vi "test Compare Labels.vi"(8 "error in":errorcluster, 11 "TestCase in":refnum<class "Refresh.lvclass">) -> (0 "error out":errorcluster, 3 "TestCase out":refnum<class "Refresh.lvclass">)   [LabVIEW 2020, in "Refresh.lvclass"]
uses:
  Refresh.lvclass
  <vilib>/addons/_JKI Toolkits/VI Tester/TestCase.llb/TestCase.lvclass
  Encoding and Decoding/Encoding.ctl
  Encoding and Decoding/Encoding and Decoding.lvlib
  Shared/Parameter Definition.ctl
  Shared/VS Channel Definition for Parameter.ctl
  System Explorer/Implementation/System Explorer/Types/Refresh Symbols.ctl
  System Explorer/Implementation/Implementation.lvlib
  System Explorer/Implementation/System Explorer/Types/Refresh Listbox.ctl
  Shared/Transfer Type.ctl
  Shared/VS Channels Definition for Label.ctl
  C:/Program Files (x86)/National Instruments/LabVIEW 2020/vi.lib/addons/_JKI Toolkits/VI Tester/TestCase.llb/TestCase.lvclass
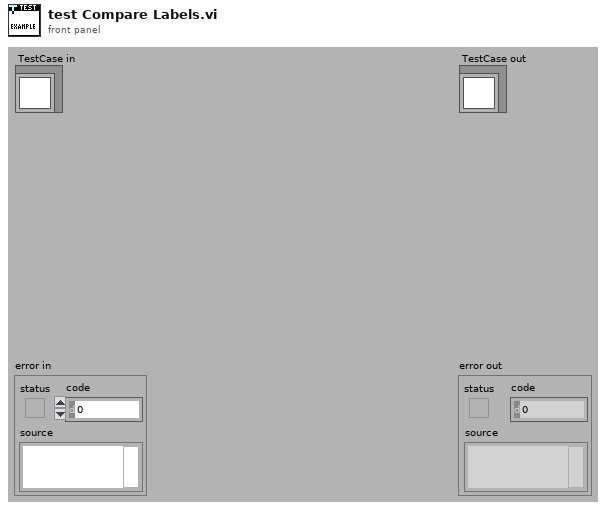
[diagram p1: front panel]
types:
  T1 = typedef "Ballard ARINC 429 System Explorer.lvlib/Implementation.lvlib/Refresh Listbox.ctl" = cluster{"Item Names":string[], "Item Symbol":T2, "Change Flag":bool}
  T2 = typedef "Ballard ARINC 429 System Explorer.lvlib/Implementation.lvlib/Refresh Symbols.ctl" = enum16{"Blank", "Port", "Incoming", "Outgoing", "Label", "Word", "Parameter", "ARINC-429", "Config Files", "Channel Spec", "Item"}
  T3 = typedef "VS Channels Definition for Label.ctl" = cluster{"label (Dec)":u32, "parameters":T4[], "SDI value":u8, "SDI enabled":bool, "transfer type":T7, "create timestamp":bool}
  T4 = typedef "VS Channel Definition for Parameter.ctl" = cluster{"name":string, "default value":dbl, "unit":string, "Parameter":T5}
  T5 = typedef "Parameter Definition.ctl" = cluster{"start index":i32, "size":i32, "encoding":T6, "signed":bool, "scale multiplier":dbl, "scale offset":dbl}
  T6 = typedef "Encoding and Decoding.lvlib/Encoding.ctl" = enum16{"BNR", "BCD", "Discrete"}
  T7 = typedef "Transfer Type.ctl" = enum16{"Scheduled", "Acyclic", "Block", "Strobe"}
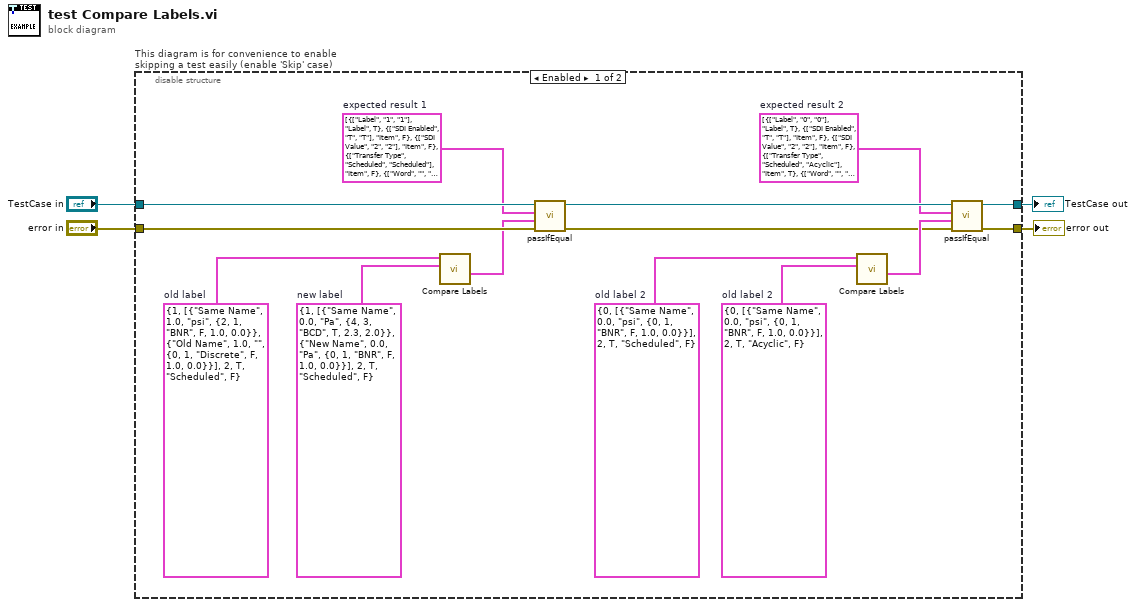
[diagram p0: block diagram]
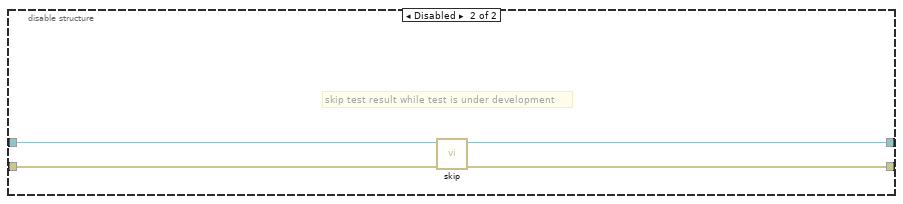
[diagram p2: hidden frame]
diagram:
  n1 = disable-structure "This diagram is for convenience to enable skipping a test easily (enable 'Skip' case)" shown="Enabled" {
    disable-tunnel: "TestCase in" -> [w18 w19]
    disable-tunnel: [w9 w20] -> w1
    disable-tunnel: [w8 w22] -> w3
    disable-tunnel: "error in" -> [w17 w21]
    frame Enabled {
      w5 = T1[] [{"Item Names"=["Label", "0", "0"], "Item Symbol"=enum."Label", "Change Flag"=TRUE}, {"Item Names"=["SDI Enabled", "TRUE", "TRUE"], "Item Symbol"=enum."Item", "Change Flag"=FALSE}, {"Item Names"=["SDI Value", "2", "2"], "Item Symbol"=enum."Item", "Change Flag"=FALSE}, {"Item Names"=["Transfer Type", "Scheduled", "Acyclic"], "Item Symbol"=enum."Item", "Change Flag"=TRUE}, {"Item Names"=["Word", "", ""], "Item Symbol"=enum."Word", "Change Flag"=FALSE}, {"Item Names"=["Parameter", "Same Name", "Same Name"], "Item Symbol"=enum."Parameter", "Change Flag"=FALSE}, {"Item Names"=["Encoding", "BNR", "BNR"], "Item Symbol"=enum."Item", "Change Flag"=FALSE}, {"Item Names"=["Default Value", "0.000000", "0.000000"], "Item Symbol"=enum."Item", "Change Flag"=FALSE}, {"Item Names"=["Start Index", "0", "0"], "Item Symbol"=enum."Item", "Change Flag"=FALSE}, {"Item Names"=["Size", "1", "1"], "Item Symbol"=enum."Item", "Change Flag"=FALSE}, {"Item Names"=["Signed", "FALSE", "FALSE"], "Item Symbol"=enum."Item", "Change Flag"=FALSE}, {"Item Names"=["Scale Factor", "1.000000", "1.000000"], "Item Symbol"=enum."Item", "Change Flag"=FALSE}, {"Item Names"=["Scale Offset", "0.000000", "0.000000"], "Item Symbol"=enum."Item", "Change Flag"=FALSE}, {"Item Names"=["Unit", "psi", "psi"], "Item Symbol"=enum."Item", "Change Flag"=FALSE}]  # expected result 2
      w7 = T3 {"label (Dec)"=0, "parameters"=[{"name"="Same Name", "default value"=0.0, "unit"="psi", "Parameter"={"start index"=0, "size"=1, "encoding"=enum."BNR", "signed"=FALSE, "scale multiplier"=1.0, "scale offset"=0.0}}], "SDI value"=2, "SDI enabled"=TRUE, "transfer type"=enum."Acyclic", "create timestamp"=FALSE}  # old label 2
      w6 = T3 {"label (Dec)"=0, "parameters"=[{"name"="Same Name", "default value"=0.0, "unit"="psi", "Parameter"={"start index"=0, "size"=1, "encoding"=enum."BNR", "signed"=FALSE, "scale multiplier"=1.0, "scale offset"=0.0}}], "SDI value"=2, "SDI enabled"=TRUE, "transfer type"=enum."Scheduled", "create timestamp"=FALSE}  # old label 2
      w13 = T1[] [{"Item Names"=["Label", "1", "1"], "Item Symbol"=enum."Label", "Change Flag"=TRUE}, {"Item Names"=["SDI Enabled", "TRUE", "TRUE"], "Item Symbol"=enum."Item", "Change Flag"=FALSE}, {"Item Names"=["SDI Value", "2", "2"], "Item Symbol"=enum."Item", "Change Flag"=FALSE}, {"Item Names"=["Transfer Type", "Scheduled", "Scheduled"], "Item Symbol"=enum."Item", "Change Flag"=FALSE}, {"Item Names"=["Word", "", ""], "Item Symbol"=enum."Word", "Change Flag"=TRUE}, {"Item Names"=["Parameter", "Same Name", "Same Name"], "Item Symbol"=enum."Parameter", "Change Flag"=TRUE}, {"Item Names"=["Encoding", "BNR", "BCD"], "Item Symbol"=enum."Item", "Change Flag"=TRUE}, {"Item Names"=["Default Value", "1.000000", "0.000000"], "Item Symbol"=enum."Item", "Change Flag"=TRUE}, {"Item Names"=["Start Index", "2", "4"], "Item Symbol"=enum."Item", "Change Flag"=TRUE}, {"Item Names"=["Size", "1", "3"], "Item Symbol"=enum."Item", "Change Flag"=TRUE}, {"Item Names"=["Signed", "FALSE", "TRUE"], "Item Symbol"=enum."Item", "Change Flag"=TRUE}, {"Item Names"=["Scale Factor", "1.000000", "2.300000"], "Item Symbol"=enum."Item", "Change Flag"=TRUE}, {"Item Names"=["Scale Offset", "0.000000", "2.000000"], "Item Symbol"=enum."Item", "Change Flag"=TRUE}, {"Item Names"=["Unit", "psi", "Pa"], "Item Symbol"=enum."Item", "Change Flag"=TRUE}, {"Item Names"=["Parameter", "", "New Name"], "Item Symbol"=enum."Parameter", "Change Flag"=TRUE}, {"Item Names"=["Encoding", "", "BNR"], "Item Symbol"=enum."Item", "Change Flag"=TRUE}, {"Item Names"=["Default Value", "", "0.000000"], "Item Symbol"=enum."Item", "Change Flag"=TRUE}, {"Item Names"=["Start Index", "", "0"], "Item Symbol"=enum."Item", "Change Flag"=TRUE}, {"Item Names"=["Size", "", "1"], "Item Symbol"=enum."Item", "Change Flag"=TRUE}, {"Item Names"=["Signed", "", "FALSE"], "Item Symbol"=enum."Item", "Change Flag"=TRUE}, {"Item Names"=["Scale Factor", "", "1.000000"], "Item Symbol"=enum."Item", "Change Flag"=TRUE}, {"Item Names"=["Scale Offset", "", "0.000000"], "Item Symbol"=enum."Item", "Change Flag"=TRUE}, {"Item Names"=["Unit", "", "Pa"], "Item Symbol"=enum."Item", "Change Flag"=TRUE}, {"Item Names"=["Parameter", "Old Name", ""], "Item Symbol"=enum."Parameter", "Change Flag"=TRUE}, {"Item Names"=["Encoding", "Discrete", ""], "Item Symbol"=enum."Item", "Change Flag"=TRUE}, {"Item Names"=["Default Value", "1.000000", ""], "Item Symbol"=enum."Item", "Change Flag"=TRUE}, {"Item Names"=["Start Index", "0", ""], "Item Symbol"=enum."Item", "Change Flag"=TRUE}, {"Item Names"=["Size", "1", ""], "Item Symbol"=enum."Item", "Change Flag"=TRUE}, {"Item Names"=["Signed", "FALSE", ""], "Item Symbol"=enum."Item", "Change Flag"=TRUE}, {"Item Names"=["Scale Factor", "1.000000", ""], "Item Symbol"=enum."Item", "Change Flag"=TRUE}, {"Item Names"=["Scale Offset", "0.000000", ""], "Item Symbol"=enum."Item", "Change Flag"=TRUE}, {"Item Names"=["Unit", "", ""], "Item Symbol"=enum."Item", "Change Flag"=TRUE}]  # expected result 1
      w14 = T3 {"label (Dec)"=1, "parameters"=[{"name"="Same Name", "default value"=1.0, "unit"="psi", "Parameter"={"start index"=2, "size"=1, "encoding"=enum."BNR", "signed"=FALSE, "scale multiplier"=1.0, "scale offset"=0.0}}, {"name"="Old Name", "default value"=1.0, "unit"="", "Parameter"={"start index"=0, "size"=1, "encoding"=enum."Discrete", "signed"=FALSE, "scale multiplier"=1.0, "scale offset"=0.0}}], "SDI value"=2, "SDI enabled"=TRUE, "transfer type"=enum."Scheduled", "create timestamp"=FALSE}  # old label
      w16 = T3 {"label (Dec)"=1, "parameters"=[{"name"="Same Name", "default value"=0.0, "unit"="Pa", "Parameter"={"start index"=4, "size"=3, "encoding"=enum."BCD", "signed"=TRUE, "scale multiplier"=2.3, "scale offset"=2.0}}, {"name"="New Name", "default value"=0.0, "unit"="Pa", "Parameter"={"start index"=0, "size"=1, "encoding"=enum."BNR", "signed"=FALSE, "scale multiplier"=1.0, "scale offset"=0.0}}], "SDI value"=2, "SDI enabled"=TRUE, "transfer type"=enum."Scheduled", "create timestamp"=FALSE}  # new label
      n2 = call "Compare Labels.vi"("new label"=w16, "old label"=w14) -> ("refresh listbox out"=w15:T1[])  [unwired: 8 in, 1 out]
      n3 = call-dynamic "passIfEqual.vi"("error in (no error)"=w17, "y"=w15, "x"=w13, "TestCase in"=w18) -> ("error out"=w10:errorcluster, "TestCase out"=w11:refnum<class "Refresh.lvclass">)  [unwired: 6 in]
      n4 = call "Compare Labels.vi"("new label"=w7, "old label"=w6) -> ("refresh listbox out"=w12:T1[])  [unwired: 8 in, 1 out]
      n5 = call-dynamic "passIfEqual.vi"("error in (no error)"=w10, "y"=w12, "x"=w5, "TestCase in"=w11) -> ("error out"=w8:errorcluster, "TestCase out"=w9:refnum<class "Refresh.lvclass">)  [unwired: 6 in]
    }
    frame Disabled {
      # "skip test result while test is under development"
      n6 = call <vilib>:"skip.vi"("error in (no error)"=w21, "TestCase in"=w19) -> ("error out"=w22:errorcluster, "TestCase out"=w20:refnum<class "Refresh.lvclass">)  [unwired: 8 in]
    }
  }
  "error out" <- w3
  "TestCase out" <- w1
